vi "Counter_V1.vi"() -> ()   [LabVIEW 2015]
panel:
  in  "Frame 2 delay":u32
  out "RPS Value":dbl
  out "time elapsed in Frame 1":u32
  out "millisecond timer value":u32
  in  "TIme per Counter Loop":u32
  in  "stop 2":bool
  out "Boolean 2":bool
  out "Sq 2 count":u8
  out "Counts":dbl
  in  "Encoder Rising Simulate":bool
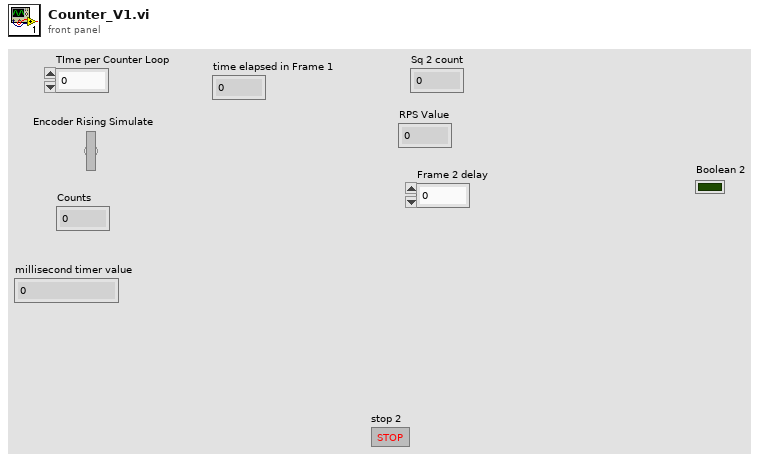
[diagram p1: front panel]
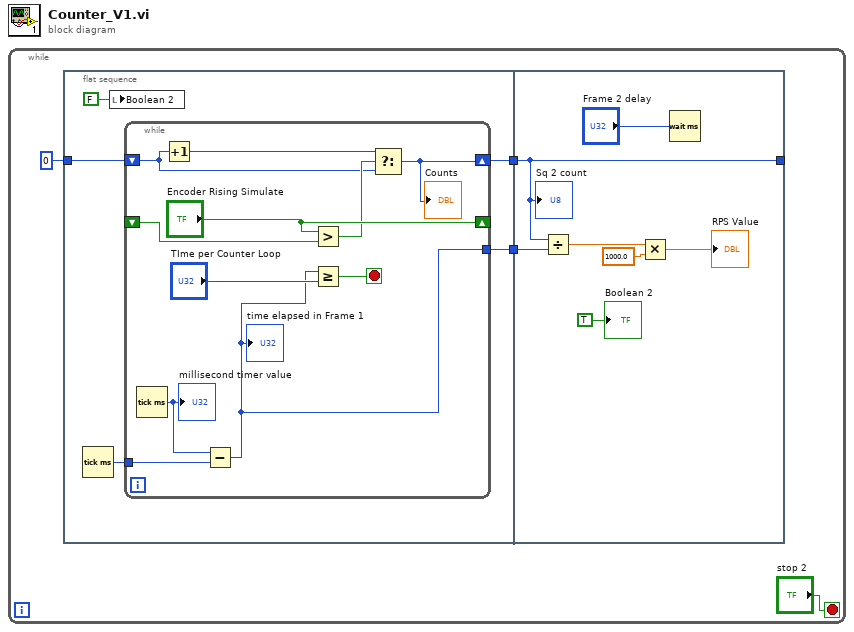
[diagram p0: block diagram]
diagram:
  n1 = while {
    stop <- "stop 2" stop-if-true
    n2 = flat-sequence {
      tunnel: [w9] -> w4
      tunnel: u8 0 -> [w7]
      tunnel: [w5] -> w1
      tunnel: w4 -> [w26]
      tunnel: [w26] -> _
      tunnel: w1 -> [w25]
      frame #0 {
        n3 = Tick Count (ms)() -> (millisecond timer value=w6:u32)
        n4 = local write "Boolean 2"(FALSE ("Boolean 2")) -> ()
        n5 = while {
          shift-right: ["Encoder Rising Simulate"] -> _
          shift-left: _ -> [w20]
          shift-right: [w15] -> w9
          shift-left: w7 -> [w16]
          tunnel: w6 -> [w12]
          tunnel: [w10] -> w5
          stop <- w14 stop-if-true
          n6 = Tick Count (ms)() -> (millisecond timer value=w13:u32)
          "millisecond timer value" <- w13
          n7 = Increment(x=w16) -> (x+1=w17:u8)
          n8 = Subtract(x=w13, y=w12) -> (x-y=w10:u32)
          "time elapsed in Frame 1" <- w10
          n9 = Greater?(x="Encoder Rising Simulate", y=w20) -> (0:w18:bool)
          n10 = Greater Or Equal?(x=w10, y="TIme per Counter Loop") -> (x >= y?=w14:bool)
          n11 = Select(t=w17, s=w18, f=w16) -> (s? t:f=w15:u8)
          "Counts" <- w15
        }
      }
      frame #1 {
        n12 = Divide(x=w26, y=w25) -> (x/y=w23:dbl)
        n13 = Multiply(x=w23, y=1000.0) -> (x*y=→"RPS Value":dbl)
        n14 = Wait (ms)(milliseconds to wait="Frame 2 delay") -> ()  [unwired: 1 out]
        "Sq 2 count" <- w26
        "Boolean 2" <- TRUE ("Boolean 2")
      }
    }
  }
